vi "Day 15-Part 2-Expand Array.vi"(11 "Array in":i32[][](array[numeric])) -> (3 "Array out":i32[][](array[numeric]))   [LabVIEW 2021]
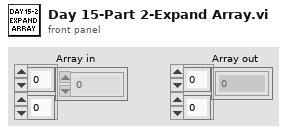
[diagram p1: front panel]
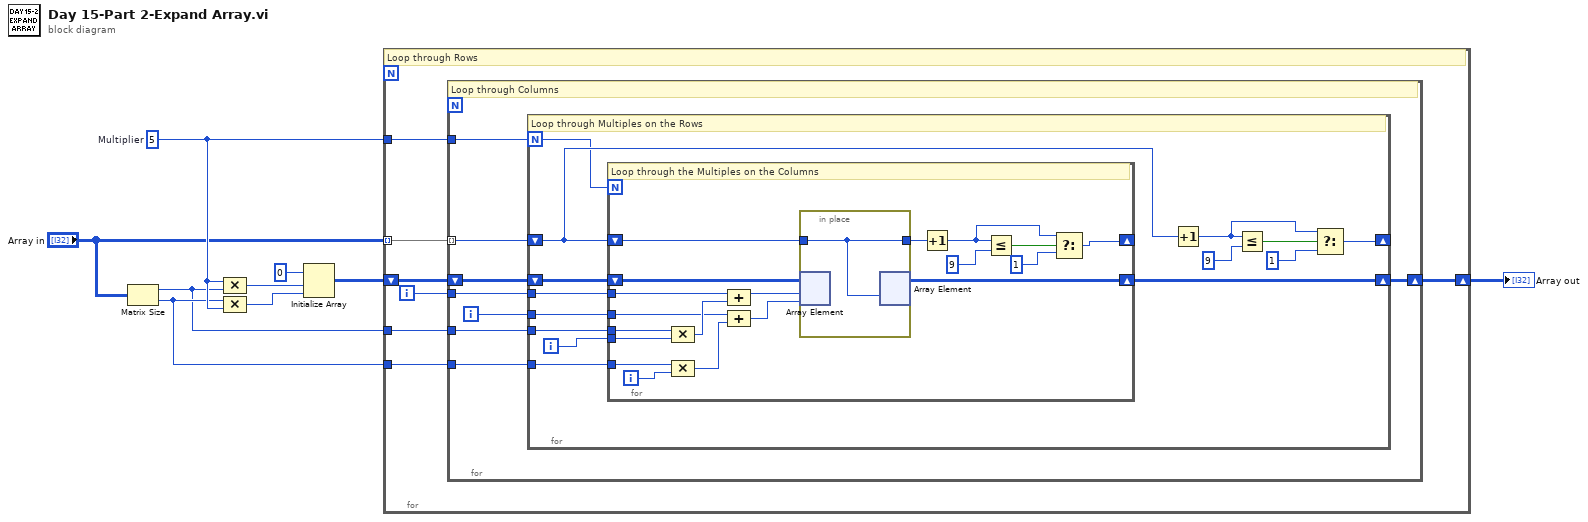
[diagram p0: block diagram]
diagram:
  w9 = 5  # Multiplier
  n1 = Matrix Size(0:"Array in") -> (1:w7:i32, 2:w8:i32)
  n2 = Compound Arithmetic op=MULTIPLY(w9, w7) -> (w3:i32)
  n3 = Compound Arithmetic op=MULTIPLY(w8, w9) -> (w5:i32)
  n4 = Initialize Array(0, w3, w5) -> (w6:i32[][])
  n5 = for {
    tunnel: "Array in" -> [w16] mode=indexing
    shift-right: [w11] -> w2
    shift-left: w6 -> [w15]
    tunnel: w7 -> [w13]
    tunnel: w8 -> [w12]
    tunnel: w9 -> [w10]
    i -> [w14]
    # "Loop through Rows"
    n6 = for {
      tunnel: w16 -> [w21] mode=indexing
      shift-right: [w18] -> w11
      shift-left: w15 -> [w24]
      tunnel: w14 -> [w23]
      tunnel: w13 -> [w20]
      tunnel: w12 -> [w19]
      tunnel: w10 -> [w17]
      i -> [w22]
      # "Loop through Columns"
      n7 = for {
        N: w17 -> [w25]
        tunnel: w23 -> [w36]
        tunnel: w22 -> [w32]
        shift-right: [w33] -> w18
        shift-left: w24 -> [w38]
        tunnel: w20 -> [w37]
        tunnel: w19 -> [w35]
        shift-right: [w28] -> _
        shift-left: w21 -> [w29]
        i -> [w34]
        # "Loop through Multiples on the Rows"
        n8 = for {
          N: w25 -> [_]
          tunnel: w37 -> [w56]
          tunnel: w36 -> [w54]
          tunnel: w35 -> [w51]
          tunnel: w34 -> [w50]
          tunnel: w32 -> [w46]
          shift-right: [w43] -> _
          shift-left: w29 -> [w48]
          shift-right: [w49] -> w33
          shift-left: w38 -> [w57]
          i -> [w42]
          # "Loop through the Multiples on the Columns"
          n9 = Compound Arithmetic op=MULTIPLY(w56, w50) -> (w55:i32)
          n10 = Compound Arithmetic op=MULTIPLY(w51, w42) -> (w52:i32)
          n11 = Compound Arithmetic op=unknown(w54, w55) -> (w53:i32)
          n12 = Compound Arithmetic op=ADD(w46, w52) -> (w41:i32)
          n13 = in-place {
            in-place-border: w48 -> [w58]
            in-place-border: [w58] -> w47
            n14 = in-place-array #1(w57, w53, w41) -> ()  [unwired: 1 out]
            n15 = in-place-array #1(w58) -> (w49:i32[][])  [unwired: 2 out]
          }
          n16 = Increment(x=w47) -> (x+1=w39:i32)
          n17 = Less Or Equal?(x=w39, y=9) -> (x <= y?=w44:bool)
          n18 = Select(t=w39, s=w44, f=1) -> (s? t:f=w43:i32)
        }
        n19 = Increment(x=w29) -> (x+1=w26:i32)
        n20 = Less Or Equal?(x=w26, y=9) -> (x <= y?=w31:bool)
        n21 = Select(t=w26, s=w31, f=1) -> (s? t:f=w28:i32)
      }
    }
  }
  "Array out" <- w2
